vi "Get Description.vi"(8 "error in (no error)":errorcluster {"code" format="Error %.0f"}, 11 "Project Documentation In":refnum<class "Project Documentation.lvclass">) -> (0 "error out":errorcluster {"code" format="Error %.0f"}, 2 "Description":string, 3 "Project Documentation Out":refnum<class "Project Documentation.lvclass">)   [LabVIEW 2023, in "VIDoc Parsing.lvlib" / "Project Documentation.lvclass"]
uses:
  Project Documentation.lvclass
  Project Documentation.lvclass/Project Documentation.ctl
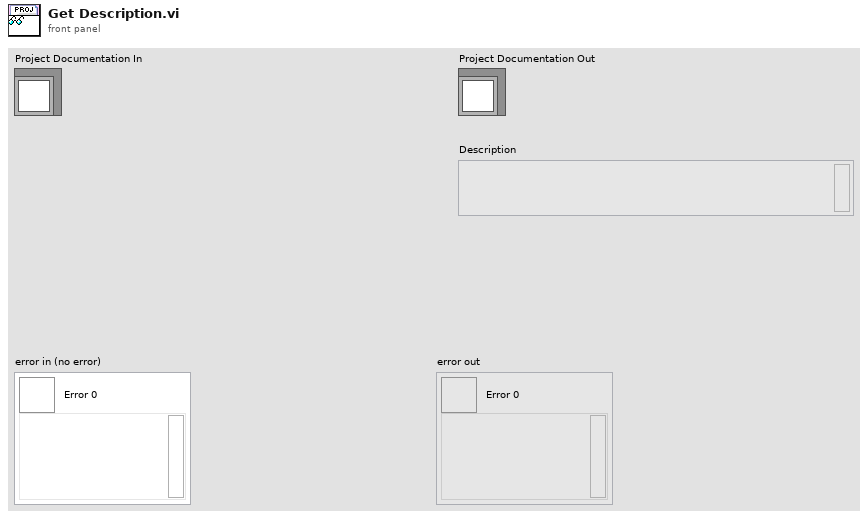
[diagram p1: front panel]
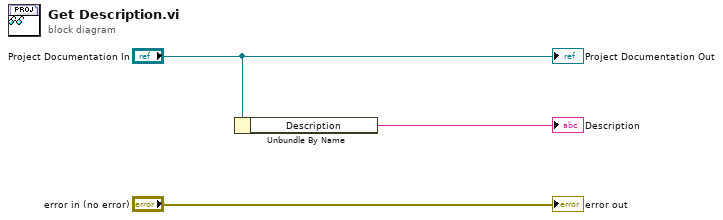
[diagram p0: block diagram]
diagram:
  n1 = Unbundle By Name("Project Documentation In") -> ("Description"=→"Description":string)
  "error out" <- "error in (no error)"
  "Project Documentation Out" <- "Project Documentation In"
